vi "Get DMA Wait Mode.vi"(8 "error in (no error)":errorcluster, 11 "Thread Configuration in":refnum<class "Thread Configuration.lvclass">) -> (0 "error out":errorcluster, 2 "wait mode":T1, 3 "Thread Configuration out":refnum<class "Thread Configuration.lvclass">)   [LabVIEW 2017, in "GE Reflective Memory.lvlib" / "Thread Configuration.lvclass"]
uses:
  Thread Configuration.lvclass
  Driver/Source/Typedefs/GE 5565PIORC.Typedef.DMA Wait Mode.ctl
  Thread Configuration.lvclass/Thread Configuration.ctl
  Driver/Source/GE 5565PIORC.lvclass
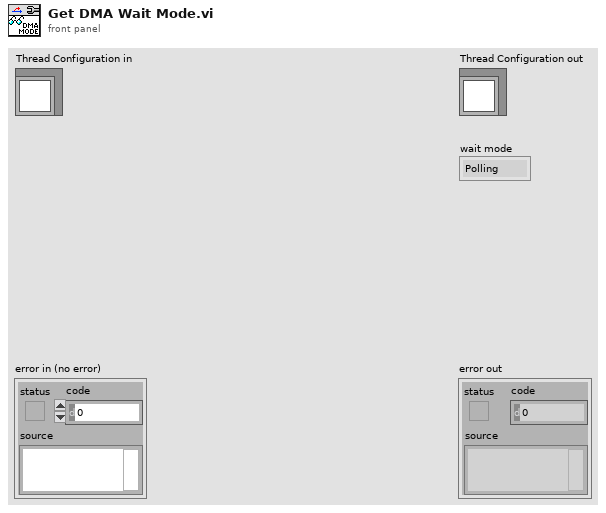
[diagram p1: front panel]
types:
  T1 = typedef "GE 5565PIORC.lvclass/GE 5565PIORC.Typedef.DMA Wait Mode.ctl" = enum16{"Polling", "Interrupt"}
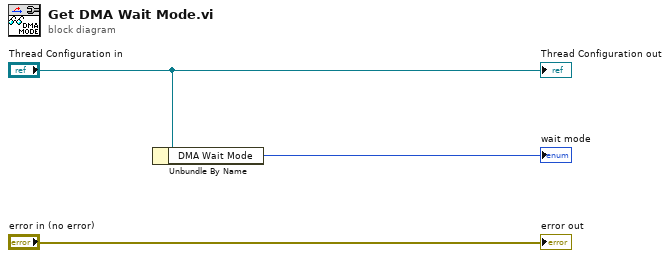
[diagram p0: block diagram]
diagram:
  n1 = Unbundle By Name("Thread Configuration in") -> ("DMA Wait Mode"=→"wait mode":T1)
  "error out" <- "error in (no error)"
  "Thread Configuration out" <- "Thread Configuration in"
